vi "Agilent 34420 Read Single.vi"() -> ()   [LabVIEW 2021]
doc: "This example shows how to configure a measurement and take a reading."
uses:
  <instrlib>/Agilent 34420/Public/Data/Read (Single Point).vi
  <instrlib>/Agilent 34420/Agilent 34420.lvlib
panel:
  in  "Function (0: DC Volts)":u16(ring) items=["DC Volts", "DC Voltage Ratio", "DC Voltage Difference", "2 Wire Resistance", "4 Wire Resistance", "Temperature"]
  out "Measurement":dbl
  in  "Serial Configuration":T1={"Baud Rate"=9600, "Parity"=0, "Data Bits"=8} {"Data Bits" items=["7"=7, "8"=8]; "Parity" items=["None", "Odd", "Even", "Mark", "Space"]; "Baud Rate" items=["300"=300, "600"=600, "1200"=1200, "2400"=2400, "4800"=4800, "9600"=9600]}
  in  "Auto Range (T: Enable)":bool=TRUE
  in  "Manual Range (0.001)":dbl=0.001
  in  "Resolution (1E-9)":dbl=1e-09
  in  "VISA resource name":refnum<visa-resource-name>
  # "(c) 2008-2015 National Instruments Corp.  ALL RIGHTS RESERVED."
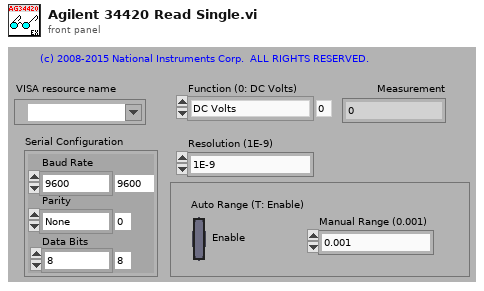
[diagram p1: front panel]
types:
  T1 = cluster{"Baud Rate":u32, "Parity":u16, "Data Bits":u16}
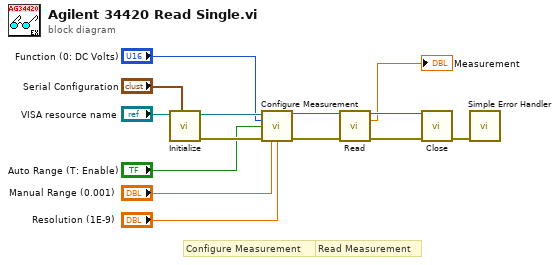
[diagram p0: block diagram]
diagram:
  # "Read Measurement"
  # "Configure Measurement"
  n1 = call <instrlib>:"Initialize.vi"("Serial Configuration"="Serial Configuration", "VISA resource name"="VISA resource name") -> ("error out"=w11:errorcluster, "VISA resource name out"=w12:refnum<visa-resource-name>)  [unwired: 8 in]
  n2 = call <instrlib>:"Configure Measurement.vi"("VISA resource name"=w12, "Function (0: DC Volts)"="Function (0: DC Volts)", "Auto Range (T:Enable)"="Auto Range (T: Enable)", "error in (no error)"=w11, "Manual Range (0.001)"="Manual Range (0.001)", "Resolution (1E-9)"="Resolution (1E-9)") -> ("VISA resource name out"=w6:refnum<visa-resource-name>, "error out"=w5:errorcluster)  [unwired: 8 in]
  n3 = call-poly <instrlib>:"Read.vi"("VISA resource name"=w6, "error in (no error)"=w5) -> ("VISA resource name out"=w7:refnum<visa-resource-name>, "Measurement"=→"Measurement":dbl, "error out"=w8:errorcluster)  [unwired: 11 in]
  n4 = call <instrlib>:"Close.vi"("error in (no error)"=w8, "VISA resource name"=w7) -> ("error out"=w14:errorcluster)  [unwired: 9 in]
  n5 = call <vilib>:"Simple Error Handler.vi"("error in (no error)"=w14) -> ()  [unwired: 4 in, 5 out]
